vi "SRV_Send No Data if Shutdown.vi"(0 "Data":string, 9 "Response Data Type":T1=enum."No Data", 11 "error in (no error)":errorcluster) -> (4 "Data dup":string, 10 "Response Data Type out":T1=enum."No Data", 15 "error out":errorcluster)   [LabVIEW 2009]
uses:
  SRV_Response Data Type.ctl
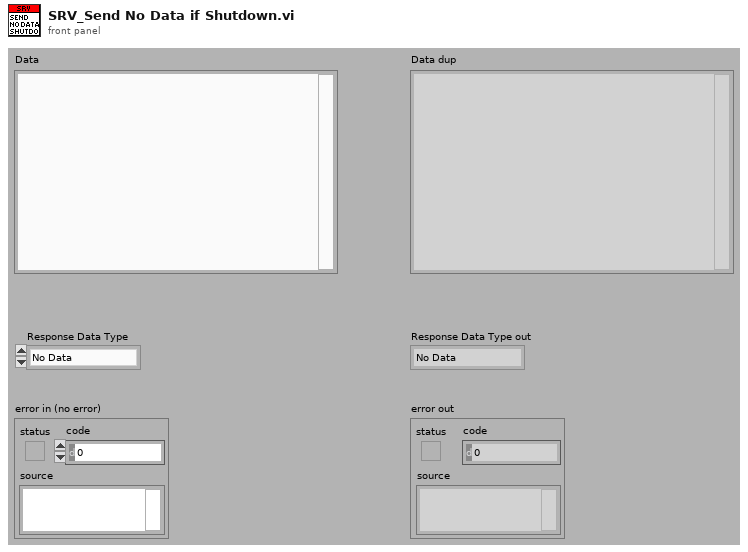
[diagram p1: front panel]
types:
  T1 = typedef "SRV_Response Data Type.ctl" = enum16{"Undefined Data", "##IMJ", "#B", "Leaving PicoC", "##vp", "##zZ", "##N$B", "##N$b", "##i$l", "##i$L", "##i$N", "##&NP,", "##&R,", "No Data"}
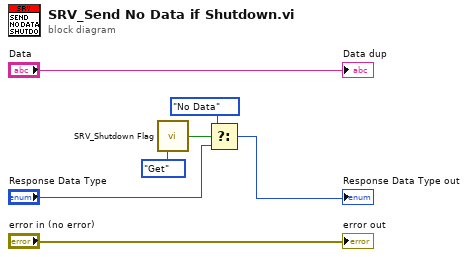
[diagram p0: block diagram]
diagram:
  n1 = call "SRV_Shutdown Flag.vi"("Method (Get)"=enum16{"Get", "Set"}."Get") -> ("Shutdown Flag out"=w6:bool)  [unwired: 13 in, 1 out]
  n2 = Select(t=SRV_Response_Data_Type."No Data" ("Response Data Type"), s=w6, f="Response Data Type") -> (s? t:f=→"Response Data Type out":T1)
  "error out" <- "error in (no error)"
  "Data dup" <- "Data"
